vi "plot_splitDisdrometer.vi"(9 "Input Arrays":dbl[][](array[numeric])=[[1.0, 4.0, 7.0], [2.0, 5.0, 8.0], [3.0, 6.0, 9.0]]) -> (10 "output cluster":T1)   [LabVIEW 2018]
doc: "Adds the datapoints for Timestamp, Rain Rate, and Accumulation to their corresponding plot arrays."
panel:
  out "Disdrometer Rain Fall":dbl[](array[numeric])
  out "Disdrometer Rain Rate":dbl[](array[numeric])
  out "Timestamp":dbl[](array[numeric])
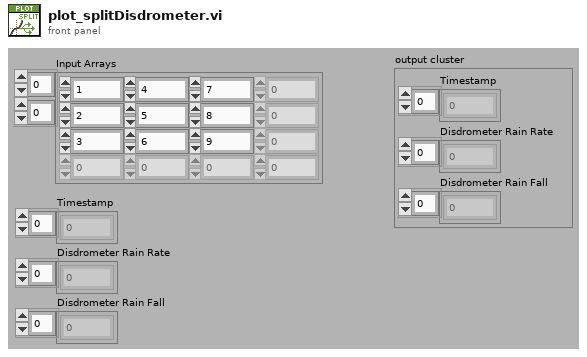
[diagram p1: front panel]
types:
  T1 = cluster{"Timestamp":dbl[], "Disdrometer Rain Rate":dbl[], "Disdrometer Rain Fall":dbl[]}
  T2 = cluster{"Input Arrays":dbl[], "Input Arrays":dbl[], "Input Arrays":dbl[]}
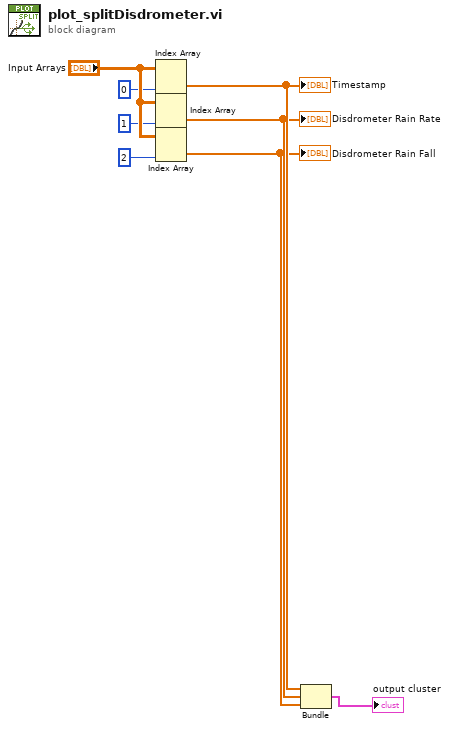
[diagram p0: block diagram]
diagram:
  n1 = Index Array(array="Input Arrays", index (col)=0 ("disabled index (col)")) -> (element=w4:dbl[])  [unwired: 1 in]
  "Timestamp" <- w4
  n2 = Index Array(array="Input Arrays", index (col)=1 ("disabled index (col)")) -> (element=w3:dbl[])  [unwired: 1 in]
  "Disdrometer Rain Rate" <- w3
  n3 = Index Array(array="Input Arrays", index (col)=2 ("disabled index (col)")) -> (element=w2:dbl[])  [unwired: 1 in]
  "Disdrometer Rain Fall" <- w2
  n4 = Bundle("Input Arrays"=w4, "Input Arrays"=w3, "Input Arrays"=w2) -> (→"output cluster":T2)  [unwired: 1 out]
